vi "Axis max.vi"(11 "Axis":dbl) -> (3 "Axis max":dbl)   [LabVIEW 2014]
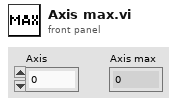
[diagram p1: front panel]
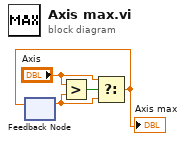
[diagram p0: block diagram]
diagram:
  n1 = feedback #1() -> (w4:dbl)  [unwired: 1 in]
  n2 = Greater?(x="Axis", y=w4) -> (0:w2:bool)
  n3 = Select(t="Axis", s=w2, f=w4) -> (s? t:f=w1:dbl)
  "Axis max" <- w1
  n4 = feedback-in #1(w1) -> ()
